vi "GetSubscriberConnections.vi"(3 "Err in":string, 4 "Response":T2, 5 "ROS registered":T4={"topic port"=0, "Node"="", "topic"="", "type"="", "node port"=0, "error "={"status"=FALSE, "code"=0, "source"=""}, "Direction"=enum."Node", "APIs"=[], "Update (ms)"=1, "write queue"=1}) -> (0 "Err out":string, 1 "Subscriber Connections":T3(array[cluster]), 2 "Logs out":T1[](array[typedef]))   [LabVIEW 2012]
uses:
  SubVIs/_ROSDirection.ctl
  SubVIs/_ROSControl.ctl
  requestTopic.ctl
  ROSLog.ctl
  _ROSDefinition.vi
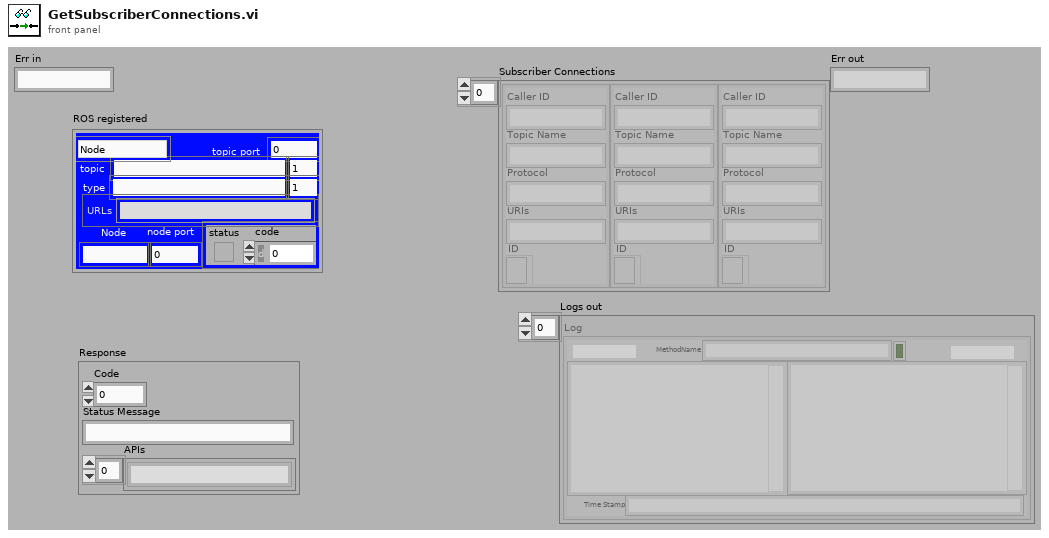
[diagram p1: front panel]
types:
  T1 = typedef "ROSLog.ctl" = cluster{"Sent":string, "Reply":string, "MethodName":string, "success":bool, "Dir1":string, "Dir2":string, "Time Stamp":string}
  T2 = cluster{"Code":i32, "Status Message":string, "APIs":string[]}
  T3 = cluster{"Caller ID":string, "Topic Name":string, "Protocol":string, "URIs":string, "ID":refnum<k5>}[]
  T4 = typedef "_ROSControl.ctl" = cluster{"topic port":u16, "Node":string, "topic":string, "type":string, "node port":u32, "error ":errorcluster, "Direction":T5, "APIs":string[], "Update (ms)":u16, "write queue":u16}
  T5 = typedef "_ROSDirection.ctl" = enum16{"Node", "Publisher", "Subscriber", "Service Client"}
  T6 = typedef "requestTopic.ctl" = cluster{"New Subscriber":cluster{"Caller ID":string, "Topic Name":string, "Protocol":string, "URIs":string, "ID":refnum<k5>}, "ROS of Server":T4, "new port":u16}
  T7 = cluster{"Caller ID":string, "Topic Name":string, "Protocol":string, "URIs":string, "ID":refnum<k5>}
  T8 = cluster{"Protocol":string, "Code":i32, "IP":string, "Port":i32}
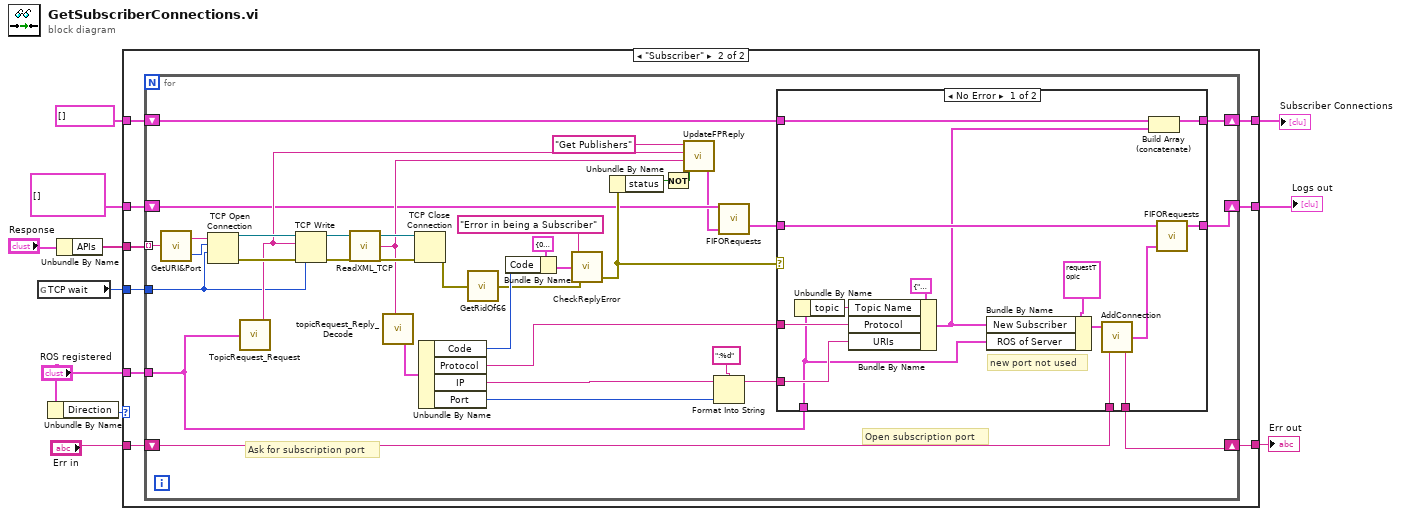
[diagram p0: block diagram]
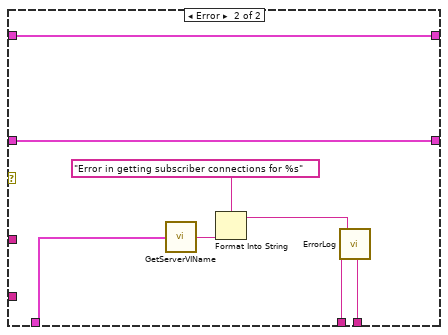
[diagram p3: hidden frame]
diagram:
  n1 = global read "_ROSDefinition.vi" "TCP wait"() -> (w3:i32)
  n2 = Unbundle By Name("ROS registered") -> ("Direction"=w4:T5)
  n3 = Unbundle By Name("Response") -> ("APIs"=w10:string[])
  n4 = case shown="\"Subscriber\"" w4 {
    tunnel: w10 -> [_ w23]
    tunnel: [w14 w22] -> w9
    tunnel: [w13 w21] -> w8
    tunnel: T3 [] ("Subscribers in") -> [w14 w20]
    tunnel: T1[] [] -> [w13 w19]
    tunnel: "ROS registered" -> [_ w18]
    tunnel: w3 -> [_ w17]
    tunnel: "Err in" -> [w12 w16]
    tunnel: [w12 w15] -> w1
    frame Default {
    }
    frame "Subscriber" {
      n5 = for {
        tunnel: w23 -> [w41] mode=indexing
        shift-right: [w39] -> w22
        shift-left: w20 -> [w40]
        shift-right: [w38] -> w21
        shift-left: w19 -> [w30]
        tunnel: w18 -> [w37]
        tunnel: w17 -> [w27]
        shift-right: [w25] -> w15
        shift-left: w16 -> [w26]
        # "Open subscription port"
        # "Ask for subscription port"
        n6 = call "GetURI&Port.vi"("URI in"=w41) -> ("Port"=w60:u16, "URI"=w59:string)
        n7 = TCP Open Connection(address=w59, remote port or service name=w60, timeout ms (60000)=w27) -> (connection ID=w43:refnum<k5>, error out=w42:errorcluster)  [unwired: 2 in]
        n8 = call "TopicRequest_Request.vi"("ROS"=w37) -> ("XML"=w35:string)
        n9 = TCP Write(connection ID=w43, data in=w35, error in (no error)=w42, 9:w27) -> (connection ID out=w44:refnum<k5>, error out=w45:errorcluster)  [unwired: 1 out]
        n10 = call "ReadXML_TCP.vi"("error in"=w45, "connection ID in"=w44) -> ("error out"=w47:errorcluster, "data out"=w34:string, "connection ID out"=w46:refnum<k5>)  [unwired: 1 in]
        n11 = call "topicRequest_Reply_Decode.vi"("Topic Request Reply"=w34) -> ("Topic Request Reply"=w48:T8)
        n12 = TCP Close Connection(connection ID=w46, error in (no error)=w47) -> (error out=w49:errorcluster)  [unwired: 1 in, 1 out]
        n13 = Unbundle By Name(w48) -> ("Code"=w56:i32, "Protocol"=w51:string, "IP"=w53:string, "Port"=w24:i32)
        n14 = call "GetRidOf66.vi"("error in (no error)"=w49) -> ("error out"=w55:errorcluster)
        n15 = Bundle By Name(cluster=T2 {"Code"=0, "Status Message"="", "APIs"=[]} ("Response"), "Code"=w56) -> (w58:T2)
        n16 = call "CheckReplyError.vi"("error in"=w55, "Response"=w58, "Error String"="Error in being a Subscriber" ("source")) -> ("error out"=w32:errorcluster)  [unwired: 2 out]
        n17 = Unbundle By Name(w32) -> ("status"=w33:bool)
        n18 = Not(x=w33) -> (.not. x?=w31:bool)
        n19 = call "UpdateFPReply.vi"("success?"=w31, "Reply"=w34, "Sent"=w35, "method"="Get Publishers") -> ("Log"=w28:T1)
        n20 = Format Into String(format string=":%d", initial string=w53, w24) -> (resulting string=w52:string)  [unwired: 1 in, 1 out]
        n21 = call "FIFORequests.vi"("Log"=w28, "Requests in"=w30) -> ("Requests out"=w29:T1[])  [unwired: 1 in]
        n22 = case shown="No Error" w32 {
          tunnel: w51 -> [w75 _]
          tunnel: w52 -> [w74 _]
          tunnel: w29 -> [w67 w83]
          tunnel: [w65 w83] -> w38
          tunnel: [w73 w82] -> w39
          tunnel: w37 -> [w61 w76]
          tunnel: w40 -> [w72 w82]
          tunnel: w26 -> [w64 w81]
          tunnel: [w63 w80] -> w25
          frame No Error {
            # "new port not used"
            n23 = Unbundle By Name(w61) -> ("topic"=w70:string)
            n24 = Bundle By Name(cluster=T7 {"Caller ID"="", "Topic Name"="", "Protocol"="", "URIs"="", "ID"=refnum} ("Subscriber"), "Topic Name"=w70, "Protocol"=w75, "URIs"=w74) -> (w62:T7)
            n25 = Bundle By Name(cluster=T6 {"New Subscriber"={"Caller ID"="", "Topic Name"="", "Protocol"="", "URIs"="", "ID"=refnum}, "ROS of Server"={"topic port"=0, "Node"="", "topic"="", "type"="", "node port"=0, "error "={"status"=FALSE, "code"=0, "source"=""}, "Direction"=enum."Node", "APIs"=[], "Update (ms)"=0, "write queue"=0}, "new port"=0} ("data"), "New Subscriber"=w62, "ROS of Server"=w61) -> (w68:T6)
            n26 = call "AddConnection.vi"("String in"=w64, "data"=w68) -> ("String out"=w63:string, "Log"=w66:T1)  [unwired: 1 in, 1 out]
            n27 = Build Array (concatenate)(w72, w62) -> (w73:T3)
            n28 = call "FIFORequests.vi"("Log"=w66, "Requests in"=w67) -> ("Requests out"=w65:T1[])  [unwired: 1 in]
          }
          frame Error {
            n29 = call "GetServerVIName.vi"("ROS"=w76) -> ("vi name"=w77:string)
            n30 = Format Into String(format string="Error in getting subscriber connections for %s" ("Error String"), w77) -> (resulting string=w78:string)  [unwired: 2 in, 1 out]
            n31 = call "ErrorLog.vi"("String in"=w81, "Error String"=w78) -> ("String out"=w80:string)  [unwired: 1 in, 1 out]
          }
        }
      }
    }
  }
  "Subscriber Connections" <- w9
  "Logs out" <- w8
  "Err out" <- w1
